vi "Cursors.vi"(6 "Cursor2 Magnitude":dbl, 7 "Cursor2 Time":dbl, 8 "error in":errorcluster, 9 "Cursor1 Magnitude":dbl, 10 "Cursor1 Time":dbl, 11 "Instrument Handle In":i32) -> (0 "error out":errorcluster, 3 "Instrument Handle Out":i32)   [LabVIEW 8.6, in "ZTScopeM.lvlib"]
doc: "Configure the cursors' positions."
uses:
  ZTScopeM.lvlib
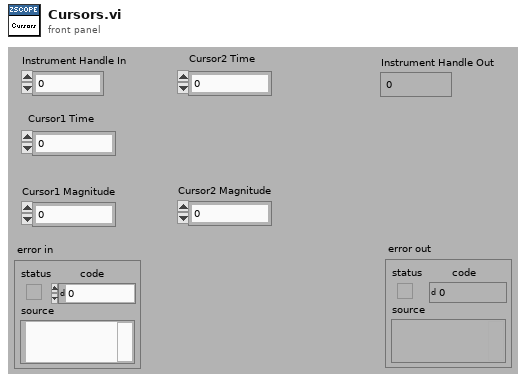
[diagram p1: front panel]
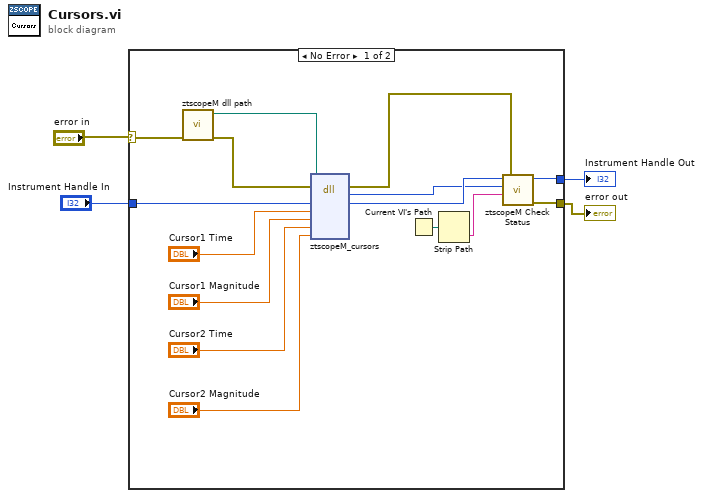
[diagram p0: block diagram]
diagram:
  n1 = case shown="No Error" "error in" {
    selector: "error in" -> [w8 w21]
    tunnel: [w10 w21] -> w1
    tunnel: "Instrument Handle In" -> [w19 w20]
    tunnel: [w9 w20] -> w3
    frame #0 {
      n2 = call "ztscopeM dll path.vi"("error in (no error)"=w8) -> ("error out"=w6:errorcluster, "<instrument>.dll path"=w7:path)  [unwired: 9 in]
      n3 = dll-call lib="C:/Program Files (x86)/National Instruments/LabVIEW 2013/instr.lib/ztscopem/ztscopeM.dll" fn="ztscopeM_cursors"(path in=w7, error in=w6, "instrumentHandle"=w19, "cursor1Time"="Cursor1 Time", "cursor1Magnitude"="Cursor1 Magnitude", "cursor2Time"="Cursor2 Time", "cursor2Magnitude"="Cursor2 Magnitude") -> (error out=w5:errorcluster, w11:i32, "instrumentHandle"=w12:i32)  [unwired: 5 in, 1 out]
      n4 = Current VI's Path() -> (path=w14:path)
      n5 = Strip Path(path=w14) -> (name=w13:string)  [unwired: 1 out]
      n6 = call "ztscopeM Check Status.vi"("error in"=w5, "name of VI"=w13, "status (return code)"=w11, "instrument handle in"=w12) -> ("error out"=w10:errorcluster, "instrument handle out"=w9:i32)  [unwired: 2 in]
    }
    frame #1 {
    }
  }
  "Instrument Handle Out" <- w3
  "error out" <- w1
